vi "iRobot Drive Radius.vi"(8 "error in":errorcluster, 9 "Radius (mm)":i16, 10 "Velocity (mm/s)":i16, 11 "UART port in":T1) -> (0 "error out":errorcluster, 3 "UART port out":T1)   [LabVIEW 2010]
doc: "Drive the robot with a fixed linear speed, and turning through a fixed radius.\n\nDo not call this VI for the special cases of driving straight, or clockwise and counter-clockwise turning; this VI instructs the robot to drive only nonzero radii.\n\nThis VI writes to, but does not read from, the serial port."
uses:
  UART/UART Port Type.ctl
  Open Interface Controls/iRobot OpCode.ctl
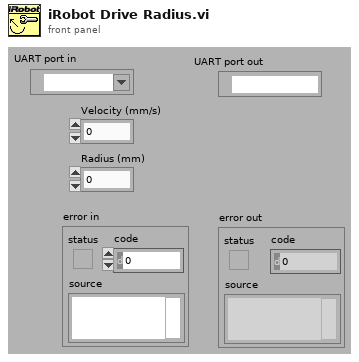
[diagram p1: front panel]
types:
  T1 = typedef "UART Port Type.ctl" = refnum<visa-resource-name>
  T2 = typedef "iRobot OpCode.ctl" = u8
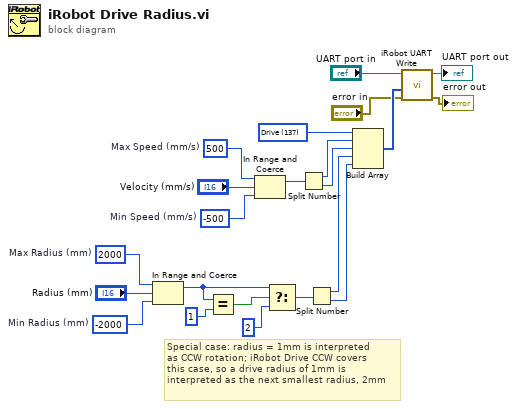
[diagram p0: block diagram]
diagram:
  w16 = i16 -2000  # Min Radius (mm)
  w15 = i16 2000  # Max Radius (mm)
  w20 = i16 -500  # Min Speed (mm/s)
  w21 = i16 500  # Max Speed (mm/s)
  w11 = T2 137 items=["Start"=128, "Baud"=129, "Control"=130, "Safe"=131, "Full"=132, "Demo"=136, "Demo - Cover"=135, "Demo - Cover and Dock"=143, "Demo - Spot"=134, "Drive"=137, "Drive Direct"=145, "LEDs"=139, "Digital Outputs"=147, "PWM Low Side Drivers"=144, "Low Side Drivers"=138, "Send IR"=151, "Song"=140, "Play Song"=141, "Sensors"=142, "Query List"=149, "Stream"=148, "Pause/Resume Stream"=150, "Script"=152, "Play Script"=153, "Show Script"=154, "Wait Time"=155, "Wait Distance"=156, "Wait Angle"=157, "Wait Event"=158] ("OpCode")
  # "Special case: radius = 1mm is interpreted\nas CCW rotation; iRobot Drive CCW covers\nthis case, so a drive radius of 1mm is\ninterpreted as the next smallest radius, 2mm"
  n1 = In Range and Coerce(upper limit=w15, x="Radius (mm)", lower limit=w16) -> (coerced(x)=w8:i16)  [unwired: 1 out]
  n2 = Equal?(x=w8, y=i16 1) -> (x = y?=w9:bool)
  n3 = In Range and Coerce(upper limit=w21, x="Velocity (mm/s)", lower limit=w20) -> (coerced(x)=w19:i16)  [unwired: 1 out]
  n4 = Select(t=w8, s=w9, f=i16 2) -> (s? t:f=w6:i16)
  n5 = Split Number(x=w19) -> (hi(x)=w18:u8, lo(x)=w17:u8)
  n6 = Split Number(x=w6) -> (hi(x)=w13:u8, lo(x)=w12:u8)
  n7 = Build Array(w11, w18, w17, w13, w12) -> (w5:T2[])
  n8 = call "iRobot UART Write.vi"("error in"="error in", "data"=w5, "UART port in"="UART port in") -> ("error out"=→"error out":errorcluster, "UART port out"=→"UART port out":T1)  [unwired: 7 in]
